vi "Send ADC.vi"(8 "error in (no error)":errorcluster, 9 "VISA resource name":refnum<visa-resource-name>, 10 "Channel ADC":u16, 11 "NXP in":refnum<class "NXP.lvclass">) -> (0 "error out":errorcluster, 1 "ADC Value":dbl, 2 "VISA resource name 2":refnum<visa-resource-name>, 3 "NXP out":refnum<class "NXP.lvclass">, 4 "concatenated string 2":string)   [LabVIEW 2020, in "NXP.lvclass"]
uses:
  NXP.lvclass
panel:
  out "concatenated string":string
  out "String 2":string
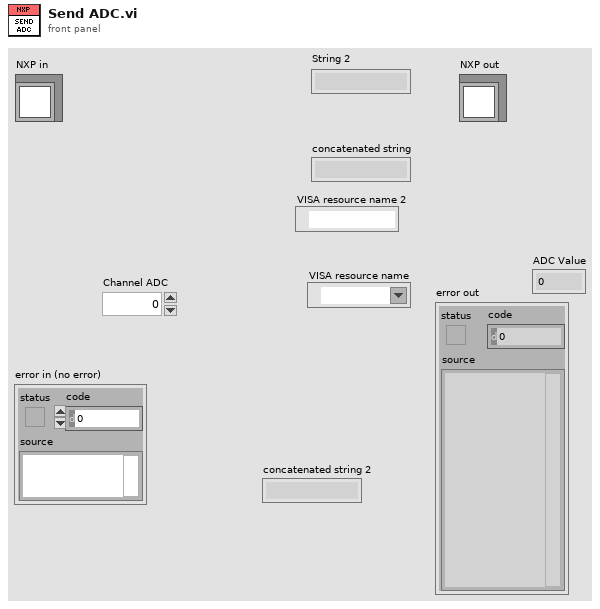
[diagram p1: front panel]
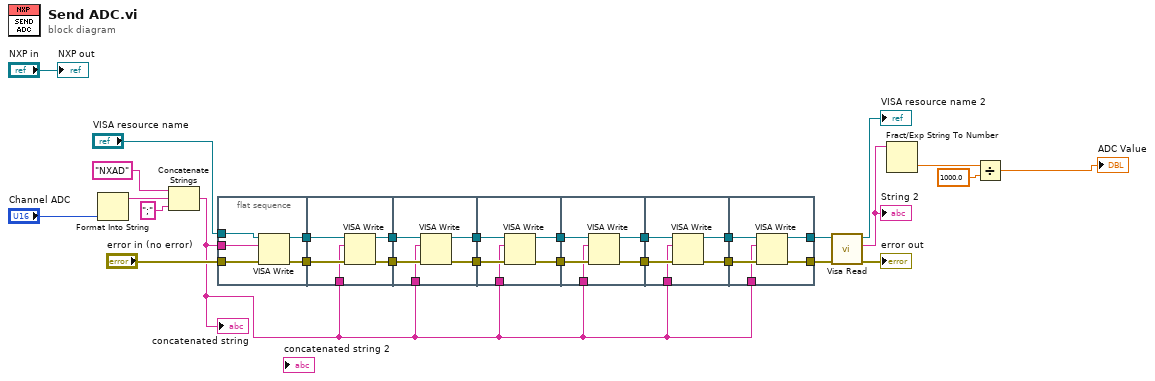
[diagram p0: block diagram]
diagram:
  n1 = Format Into String("Channel ADC") -> (resulting string=w27:string)  [unwired: 3 in, 1 out]
  n2 = Concatenate Strings("NXAD" ("string"), w27, ";" ("string")) -> (w4:string)
  "concatenated string" <- w4
  n3 = flat-sequence {
    tunnel: "VISA resource name" -> [w33]
    tunnel: w4 -> [w32]
    tunnel: "error in (no error)" -> [w31]
    tunnel: [w30] -> w16
    tunnel: [w29] -> w15
    tunnel: w16 -> [w38]
    tunnel: w15 -> [w37]
    tunnel: [w36] -> w14
    tunnel: [w35] -> w13
    tunnel: w4 -> [w34]
    tunnel: w14 -> [w43]
    tunnel: w13 -> [w42]
    tunnel: [w41] -> w12
    tunnel: [w40] -> w11
    tunnel: w4 -> [w39]
    tunnel: w12 -> [w48]
    tunnel: w11 -> [w47]
    tunnel: [w46] -> w10
    tunnel: [w45] -> w9
    tunnel: w4 -> [w44]
    tunnel: w10 -> [w53]
    tunnel: w9 -> [w52]
    tunnel: [w51] -> w8
    tunnel: [w50] -> w7
    tunnel: w4 -> [w49]
    tunnel: w8 -> [w58]
    tunnel: w7 -> [w57]
    tunnel: [w56] -> w6
    tunnel: [w55] -> w5
    tunnel: w4 -> [w54]
    tunnel: w6 -> [w63]
    tunnel: w5 -> [w62]
    tunnel: w4 -> [w61]
    tunnel: [w60] -> w3
    tunnel: [w59] -> w2
    frame #0 {
      n4 = VISA Write(VISA resource name=w33, write buffer=w32, error in (no error)=w31) -> (VISA resource name out=w29:refnum<visa-resource-name>, error out=w30:errorcluster)  [unwired: 1 out]
    }
    frame #1 {
      n5 = VISA Write(VISA resource name=w37, write buffer=w34, error in (no error)=w38) -> (VISA resource name out=w36:refnum<visa-resource-name>, error out=w35:errorcluster)  [unwired: 1 out]
    }
    frame #2 {
      n6 = VISA Write(VISA resource name=w43, write buffer=w39, error in (no error)=w42) -> (VISA resource name out=w41:refnum<visa-resource-name>, error out=w40:errorcluster)  [unwired: 1 out]
    }
    frame #3 {
      n7 = VISA Write(VISA resource name=w48, write buffer=w44, error in (no error)=w47) -> (VISA resource name out=w46:refnum<visa-resource-name>, error out=w45:errorcluster)  [unwired: 1 out]
    }
    frame #4 {
      n8 = VISA Write(VISA resource name=w53, write buffer=w49, error in (no error)=w52) -> (VISA resource name out=w50:refnum<visa-resource-name>, error out=w51:errorcluster)  [unwired: 1 out]
    }
    frame #5 {
      n9 = VISA Write(VISA resource name=w57, write buffer=w54, error in (no error)=w58) -> (VISA resource name out=w56:refnum<visa-resource-name>, error out=w55:errorcluster)  [unwired: 1 out]
    }
    frame #6 {
      n10 = VISA Write(VISA resource name=w63, write buffer=w61, error in (no error)=w62) -> (VISA resource name out=w60:refnum<visa-resource-name>, error out=w59:errorcluster)  [unwired: 1 out]
    }
  }
  n11 = call "Visa Read.vi"("error in (no error)"=w2, "VISA Refnum in"=w3) -> ("error out"=→"error out":errorcluster, "String 2"=w22:string, "VISA Refnum out"=→"VISA resource name 2":refnum<visa-resource-name>)  [unwired: 7 in]
  "String 2" <- w22
  n12 = Fract/Exp String To Number(string=w22) -> (number=w21:dbl)  [unwired: 3 in, 1 out]
  n13 = Divide(x=w21, y=1000.0) -> (x/y=→"ADC Value":dbl)
  "NXP out" <- "NXP in"
